vi "getImage2Array.vi"(2 "exposureUnitsPrefix":dbl, 3 "New Image":T2, 4 "ExpsureTime":dbl, 5 "Session in":T1) -> (0 "exposureReadback":dbl, 1 "Image Array":u16[][](array[numeric]))   [LabVIEW 2021]
uses:
  <vilib>/vision/Image Controls.llb/IMAQ Image.ctl
  <vilib>/userdefined/High Color/IMAQdx.ctl
  <vilib>/vision/driver/IMAQdx.llb/IMAQdx Buffer Number Mode.ctl
  <vilib>/vision/driver/NI_Vision_Acquisition_Software.lvlib
  <resource>/objmgr/imaqdx.rc
panel:
  out "error out":errorcluster
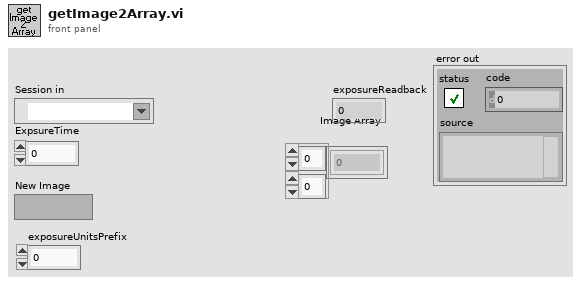
[diagram p1: front panel]
types:
  T1 = typedef "IMAQdx.ctl" = refnum<k21>
  T2 = typedef "IMAQ Image.ctl" = refnum<image>
  T3 = typedef "NI_Vision_Acquisition_Software.lvlib/IMAQdx Buffer Number Mode.ctl" = enum32{"Next", "Last", "Buffer Number", "Every", "Last New"}
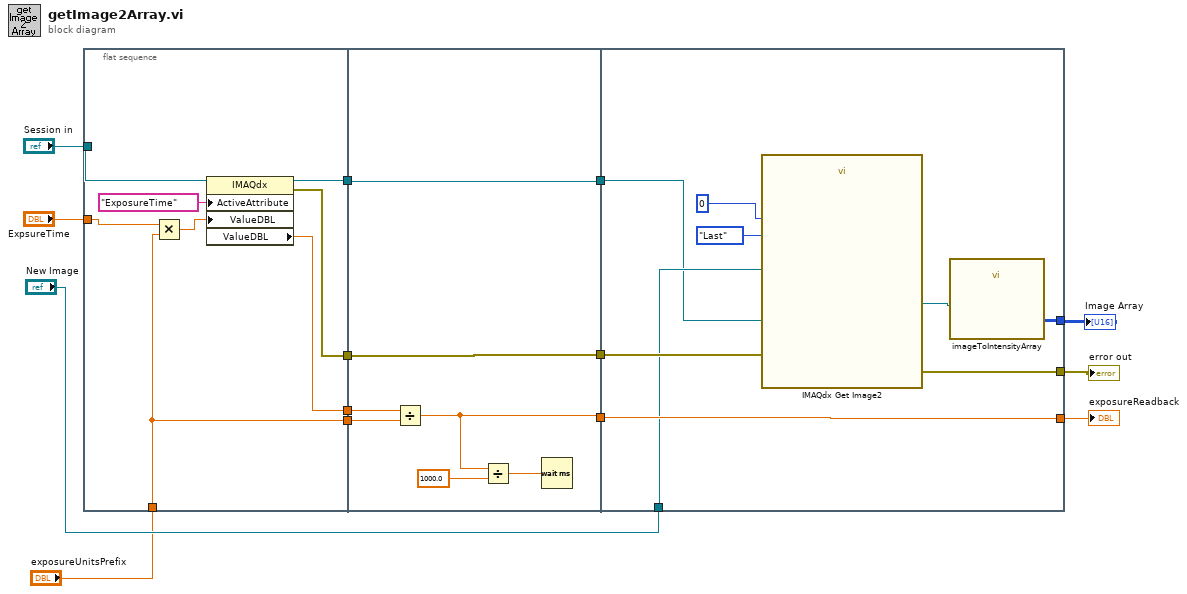
[diagram p0: block diagram]
diagram:
  n1 = flat-sequence {
    tunnel: "ExpsureTime" -> [w16]
    tunnel: "Session in" -> [w18]
    tunnel: [w22] -> w12
    tunnel: [w20] -> w11
    tunnel: [w19] -> w10
    tunnel: "exposureUnitsPrefix" -> [w15]
    tunnel: [w15] -> w1
    tunnel: w12 -> [w29]
    tunnel: w11 -> [w28]
    tunnel: w10 -> [w26]
    tunnel: [w29] -> w9
    tunnel: [w28] -> w8
    tunnel: [w24] -> w7
    tunnel: w1 -> [w23]
    tunnel: [w38] -> w4
    tunnel: w9 -> [w32]
    tunnel: w8 -> [w35]
    tunnel: w7 -> [w38]
    tunnel: "New Image" -> [w33]
    tunnel: [w31] -> w5
    tunnel: [w30] -> w3
    frame #0 {
      n2 = Multiply(x=w16, y=w15) -> (x*y=w17:dbl)
      n3 = property class="IMAQdx"(reference=w18, "ActiveAttribute"="ExposureTime", "ValueDBL"=w17) -> (reference out=w22:T1, error out=w20:errorcluster, "ValueDBL"=w19:dbl)  [unwired: 1 in]
    }
    frame #1 {
      n4 = Divide(x=w26, y=w23) -> (x/y=w24:dbl)
      n5 = Divide(x=w24, y=1000.0) -> (x/y=w27:dbl)
      n6 = Wait (ms)(milliseconds to wait=w27) -> ()  [unwired: 1 out]
    }
    frame #2 {
      n7 = call <vilib>:"IMAQdx Get Image2.vi"("Buffer Number Mode (Next)"=IMAQdx_Buffer_Number_Mode."Last", "error in"=w35, "Buffer Number In"=u32 0, "Image In"=w33, "Session In"=w32) -> ("error out"=w30:errorcluster, "Image Out"=w37:T2)  [unwired: 3 in, 2 out]
      n8 = call "imageToIntensityArray.vi"("image"=w37) -> ("imageArray"=w31:u16[][])  [unwired: 10 in]
    }
  }
  "Image Array" <- w5
  "exposureReadback" <- w4
  "error out" <- w3
